vi "production_canette.vi"(1 "Ajout sucre":bool, 2 "Pas ajout sucre":bool, 3 "?":bool, 4 "Pas ajout Gaz":bool, 5 "Ajout Gaz":bool, 6 "Radio Buttons":enum32{"Radio Selection 1", "Radio Selection 2"}(radio), 7 "StartB":bool, 8 "stop":bool) -> (0 "cannettes produites":dbl)   [LabVIEW 2023]
uses:
  selector.ctl
  Control 1.ctl
  Control 5.ctl
  <vilib>/numeric/Random Number (Range) U64.vi
  <vilib>/numeric/sub_Random U32.vi
panel:
  in  "Selector":T1
  out "Produits defectueux":dbl
  out "Produits Finis":dbl
  out "Nb cycles":dbl
  in  "fini":bool
  out "MP3 2":bool
  out "Valeur PH":dbl
  out "Boolean":bool
  in  "Seuil PH":dbl(slide) scale=0.0..14.0
  out "Tab Control":T2(tab)
  out "MP3":bool
  out "Tank":cluster{dbl, dbl}(slide)={0.0, 10.0} scale=0.0..10.0
  # "DO u want gaz ?"
  # "DO u want sugar ?"
  # "Production finie"
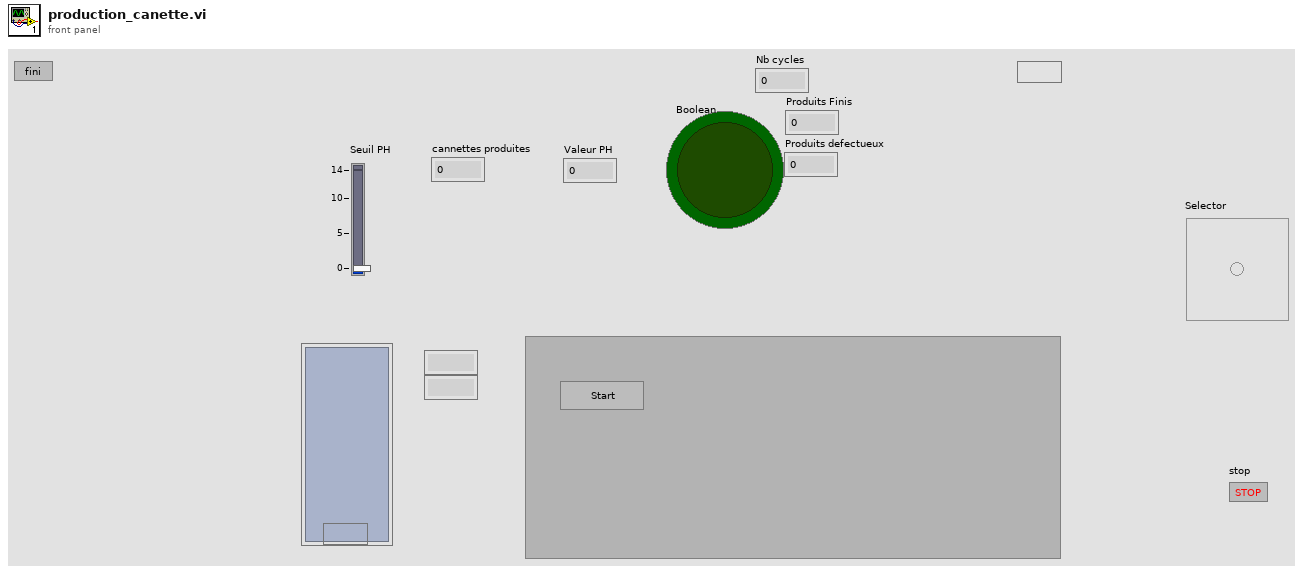
[diagram p1: front panel]
types:
  T1 = typedef "selector.ctl" = bool
  T2 = enum32{"Start", "Type", "preparer", "GazS", "GazF", "Sugar", "Finish"}
  T3 = typedef "Control 1.ctl" = enum32{"Start", "Page 1", "Page 2", "Page 3", "Page 4", "Sugar", "Finish"}
  T4 = typedef "Control 5.ctl" = enum32{"Start", "Page 1", "Page 2", "Page 3", "Page4"}
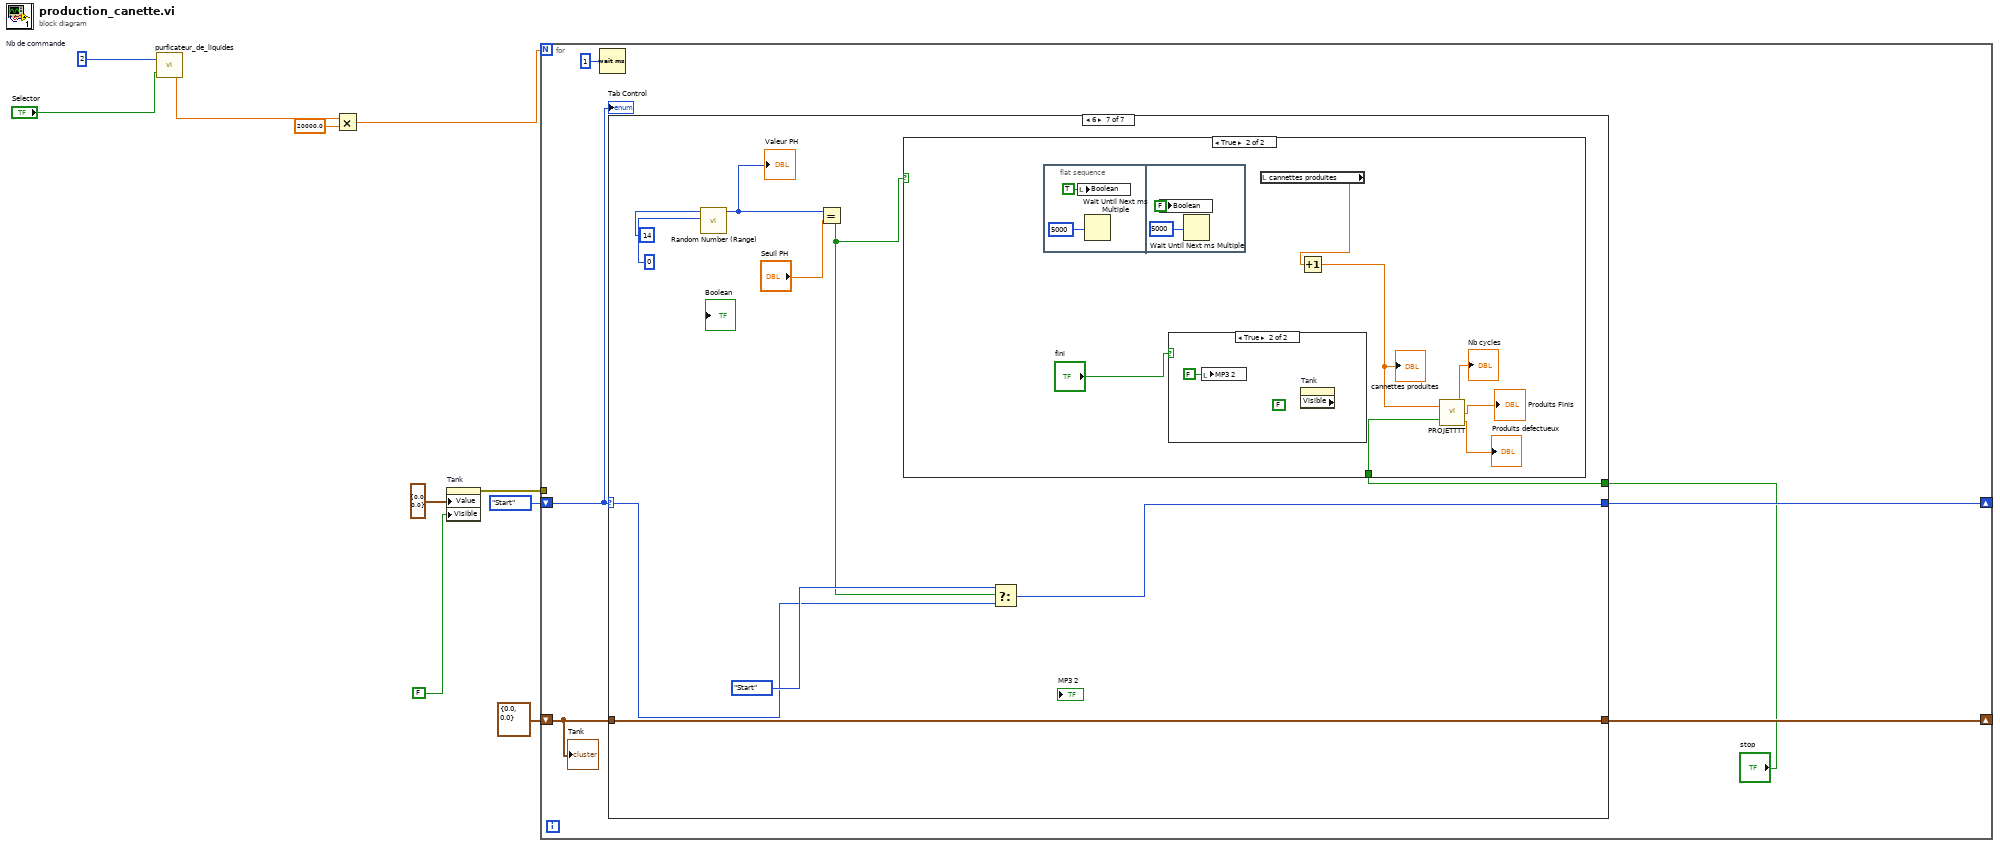
[diagram p0: block diagram]
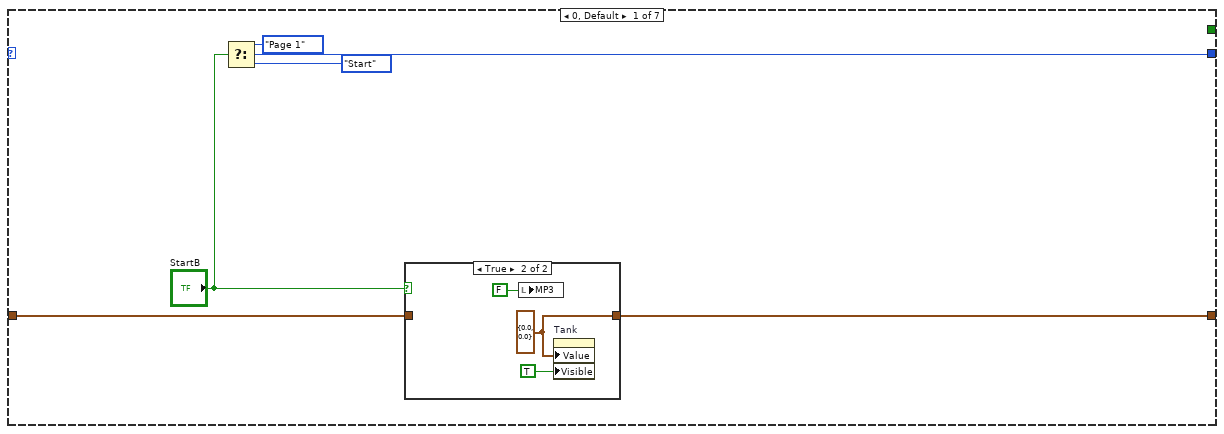
[diagram p2: hidden frame]
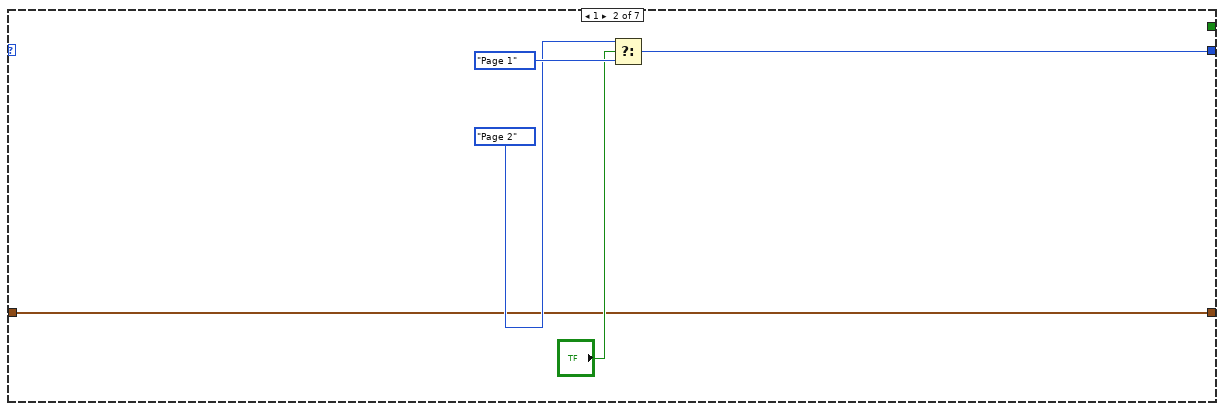
[diagram p4: hidden frame]
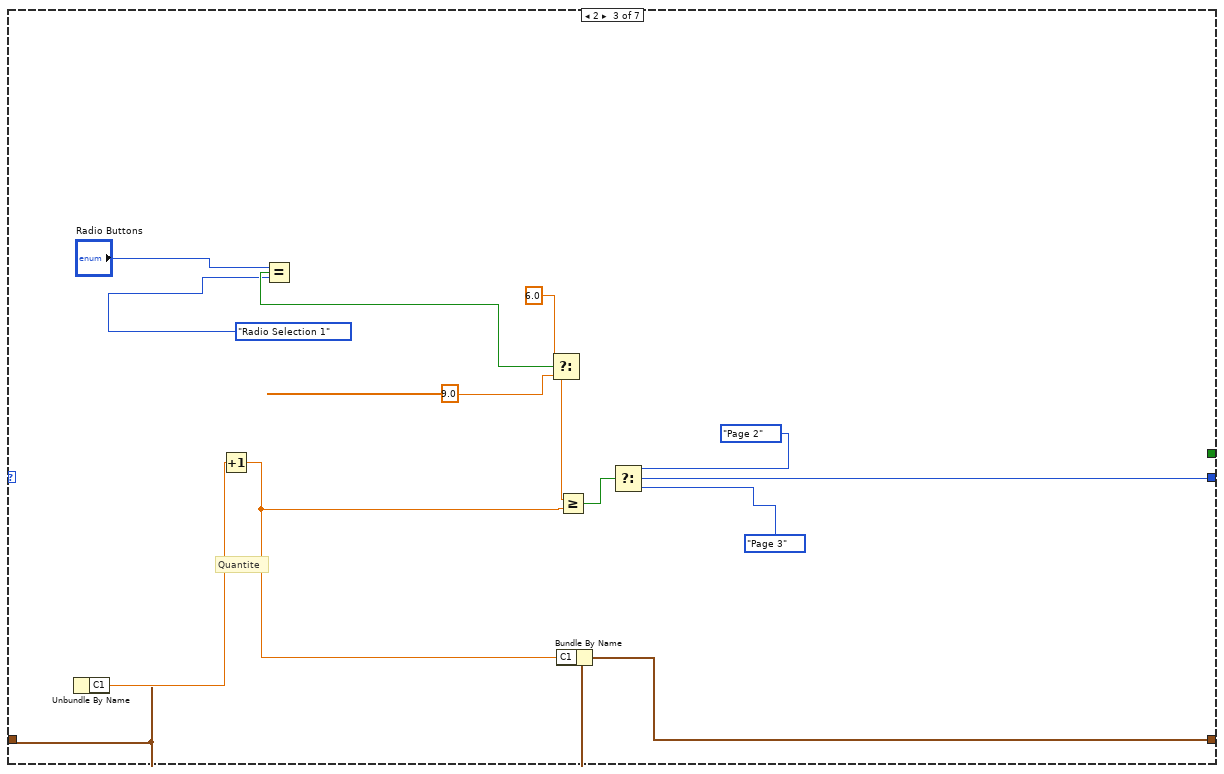
[diagram p5: hidden frame]
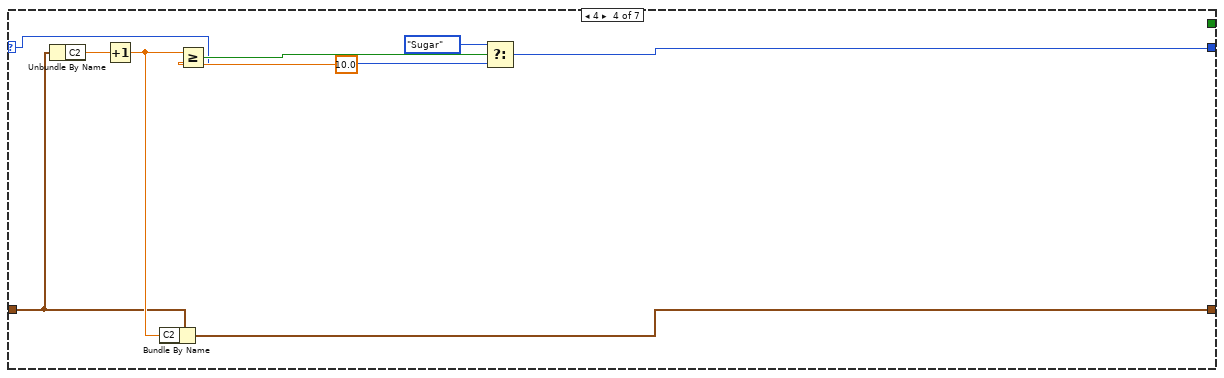
[diagram p6: hidden frame]
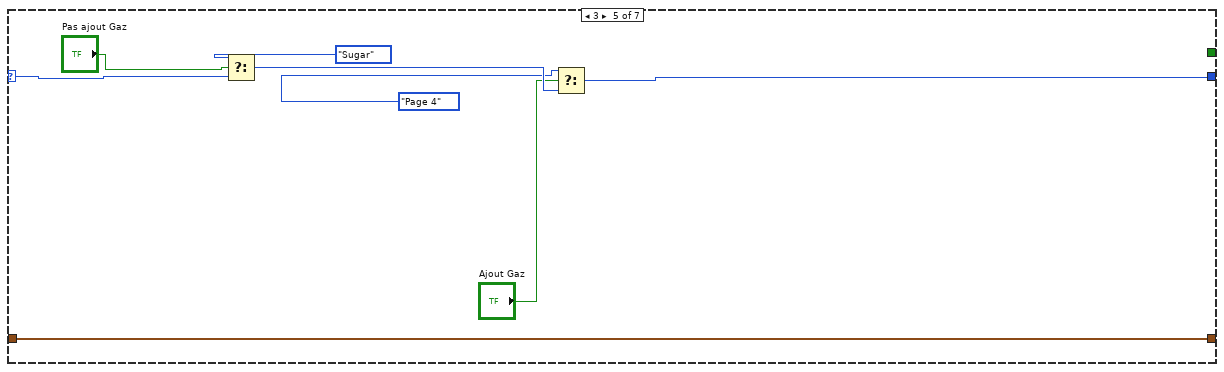
[diagram p7: hidden frame]
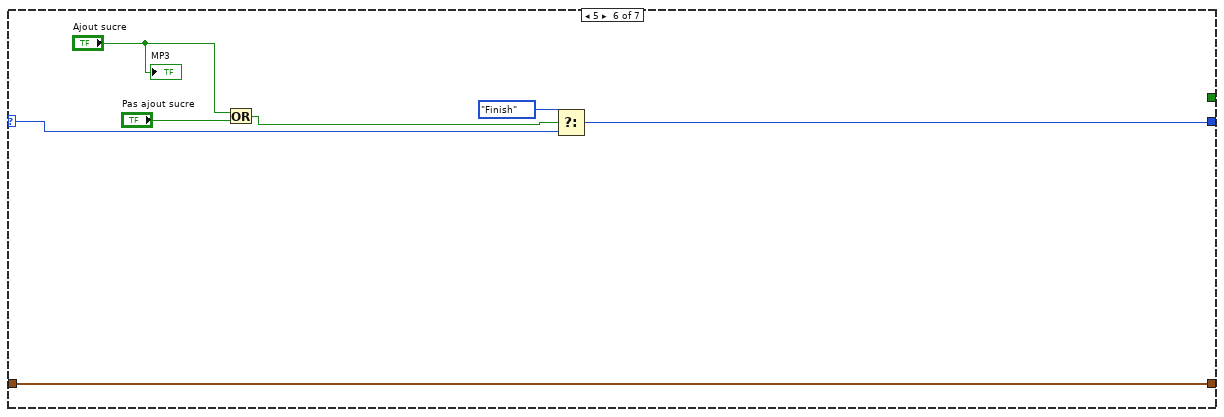
[diagram p8: hidden frame]
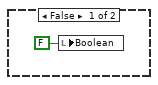
[diagram p9: hidden frame]
diagram:
  w2 = 2  # Nb de commande
  n1 = call "purficateur_de_liquides.vi"("Bouton OK 3"="Selector", "Nb de litres recus"=w2) -> ("nb de litres purifies"=w3:dbl)
  n2 = Multiply(x=w3, y=20000.0) -> (x*y=w4:dbl)
  n3 = property on="Tank" class="Slide (strict)"("Value"=cluster{dbl, dbl} {0.0, 0.0} ("Tank"), "Visible"=FALSE) -> (error out=w7:errorcluster)  [unwired: 2 in, 1 out]
  n4 = for {
    N: w4 -> [_]
    shift-right: [w16] -> _
    shift-left: cluster{"C1":dbl, "C2":dbl} {"C1"=0.0, "C2"=0.0} ("Tank") -> [w13]
    shift-right: [w14] -> _
    shift-left: Control_1."Start" ("Tab Control") -> [w15]
    tunnel: w7 -> [_]
    n5 = Wait (ms)(milliseconds to wait=u32 1 ("millisecond timer value")) -> ()  [unwired: 1 out]
    n6 = case shown="6" w15 {
      selector: w15 -> [_ _ _ w48 w61 w67 w77]
      tunnel: [w19 w28 w34 w46 w58 w64 w76] -> w14
      tunnel: w13 -> [w18 w27 w39 w50 w55 w69 w79]
      tunnel: [w17 w27 w38 w49 w55 w69 w79] -> w16
      tunnel: "stop" -> [_ _ _ _ _ _ w70]
      frame 0, Default {
        n7 = Select(t=Control_5."Page 1" ("Tab Control"), s="StartB", f=Control_5."Start" ("Tab Control")) -> (s? t:f=w19:T4)
        n8 = case shown="True" "StartB" {
          tunnel: [w23 w24] -> w17
          tunnel: w18 -> [w23 _]
          frame False {
          }
          frame True {
            w24 = cluster{dbl, dbl} {0.0, 0.0} ("Tank")
            n9 = local write "MP3"(FALSE ("MP3")) -> ()
            n10 = property on="Tank" class="Slide (strict)"("Value"=w24, "Visible"=TRUE) -> ()  [unwired: 2 in, 2 out]
          }
        }
      }
      frame 1 {
        n11 = Select(t=Control_5."Page 2" ("Tab Control"), s="?", f=Control_5."Page 1" ("Tab Control")) -> (s? t:f=w28:T4)
      }
      frame 2 {
        # "Quantite"
        n12 = Unbundle By Name(w39) -> ("C1"=w40:dbl)
        n13 = Increment(x=w40) -> (x+1=w33:dbl)
        n14 = Equal?(x="Radio Buttons", y=enum32{"Radio Selection 1", "Radio Selection 2"}."Radio Selection 1" ("x")) -> (x = y?=w43:bool)
        n15 = Select(t=6.0, s=w43, f=9.0) -> (s? t:f=w32:dbl)
        n16 = Bundle By Name(cluster=w39, "C1"=w33) -> (w38:cluster{"C1":dbl, "C2":dbl})
        n17 = Greater Or Equal?(x=w32, y=w33) -> (x >= y?=w35:bool)
        n18 = Select(t=Control_5."Page 2" ("Tab Control"), s=w35, f=Control_5."Page 3" ("Tab Control")) -> (s? t:f=w34:T4)
      }
      frame 4 {
        n19 = Unbundle By Name(w50) -> ("C2"=w54:dbl)
        n20 = Increment(x=w54) -> (x+1=w53:dbl)
        n21 = Bundle By Name(cluster=w50, "C2"=w53) -> (w49:cluster{"C1":dbl, "C2":dbl})
        n22 = Greater Or Equal?(x=w53, y=10.0) -> (x >= y?=w52:bool)
        n23 = Select(t=Control_1."Sugar" ("Tab Control"), s=w52, f=w48) -> (s? t:f=w46:u32)
      }
      frame 3 {
        n24 = Select(t=Control_1."Sugar" ("Tab Control"), s="Pas ajout Gaz", f=w61) -> (s? t:f=w60:u32)
        n25 = Select(t=Control_1."Page 4" ("Tab Control"), s="Ajout Gaz", f=w60) -> (s? t:f=w58:u32)
      }
      frame 5 {
        n26 = Or(x="Ajout sucre", y="Pas ajout sucre") -> (x .or. y?=w66:bool)
        n27 = Select(t=Control_1."Finish" ("Tab Control"), s=w66, f=w67) -> (s? t:f=w64:u32)
        "MP3" <- "Ajout sucre"
      }
      frame 6 {
        n28 = call-poly <vilib>:"Random Number (Range).vi"("lower bound (0)"=u64 0, "upper bound (100)"=u64 14) -> ("number"=w75:u64)  [unwired: 9 in]
        "Valeur PH" <- w75
        n29 = Equal?(x=w75, y="Seuil PH") -> (x = y?=w71:bool)
        n30 = case shown="True" w71 {
          tunnel: w70 -> [_ w81]
          frame False {
            n31 = local write "Boolean"(FALSE ("Boolean")) -> ()
          }
          frame True {
            n32 = flat-sequence {
              frame #0 {
                n33 = local write "Boolean"(TRUE ("Boolean")) -> ()
                n34 = Wait Until Next ms Multiple(millisecond multiple=u32 5000 ("millisecond timer value")) -> ()  [unwired: 1 out]
              }
              frame #1 {
                n35 = local write "Boolean"(FALSE ("Boolean")) -> ()
                n36 = Wait Until Next ms Multiple(millisecond multiple=u32 5000 ("millisecond timer value")) -> ()  [unwired: 1 out]
              }
            }
            n37 = case shown="True" "fini" {
              frame False {
              }
              frame True {
                (unwired) FALSE ("Visible")
                n38 = local write "MP3 2"(FALSE ("MP3")) -> ()
                n39 = property on="Tank" class="Slide (strict)" props=["Visible"]() -> ()  [unwired: 2 in, 3 out]
              }
            }
            n40 = local read "cannettes produites"() -> (w87:dbl)
            n41 = Increment(x=w87) -> (x+1=w84:dbl)
            "cannettes produites" <- w84
            n42 = call "PROJETTTT.vi"("Numérique"=w84, "stop"=w81) -> ("Nb cycles"=→"Nb cycles":dbl, "Produits Finis"=→"Produits Finis":dbl, "Produits defectueux"=→"Produits defectueux":dbl)
          }
        }
        n43 = Select(t=Control_1."Start" ("Tab Control"), s=w71, f=w77) -> (s? t:f=w76:u32)
      }
    }
    "Tab Control" <- w15
    "Tank" <- w13
  }
